vi "CSM - LogViewer2.vi"() -> ()   [LabVIEW 2017]
uses:
  Utility/_support/Periodic String Filter Level.ctl
  _jksm/_action.ctl
  Utility/Periodic String Filter Setting.ctl
  <vilib>/addons/_JKI Toolkits/State Machine/_JKI_lib_State_Machine.llb/Parse State Queue__JKI_lib_State_Machine.vi
  Communicable State Machine.lvlib
  _Shared/CSM Shared.lvlib
  _Support/csm-tool-support.lvlib
  _csmHelper/API with lvcsm Support/CSM-Helper API with lvcsm Support.lvlib
  addons/Logger/CSM File Logger.lvlib
  _ui/csm-ui-support.lvlib
  _jksm/_jkism_magic.lvlib
panel:
  out "Error(#)":i64 caption="Error(#):"
  in  "Record.Stop":bool
  in  "Record.Start":bool
  in  "Clear":bool
  in  "BackTop":bool
  in  "Toolbar.History Length(char)":i32=50000 caption="History(char)" min=1000 max=100000000 step=1
  in  "Peroid Logs":bool
  in  "Tab":T1(tab)
  out "State History":string
  out "Error History":string
  out "Broadcast Registry":string[][](table)
  out "LogInQ":i32 caption="LogInQ:"
  out "log handling Speed(#/s)":dbl caption="log handling Speed(#/s):"
  out "LogInQ change(#/s)":dbl caption="LogInQ change(#/s):"
  out "Level":T2 caption="Level:"
  in  "Stop":bool
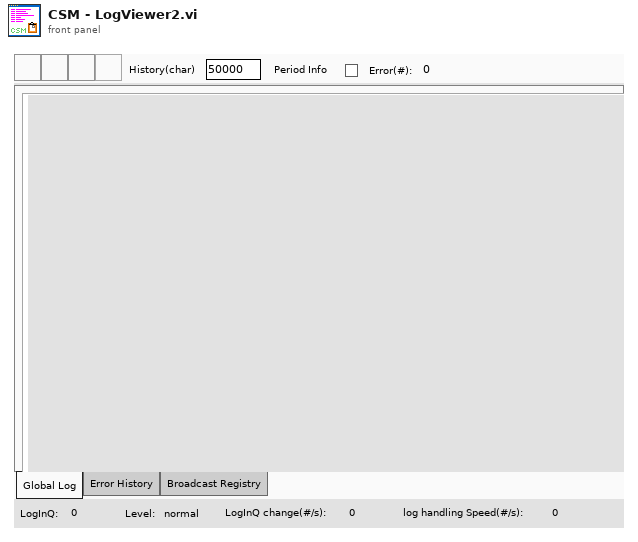
[diagram p1: front panel]
types:
  T1 = enum32{"Global Log", "Error History", "Broadcast Registry"}
  T2 = typedef "Communicable State Machine.lvlib/Periodic String Filter Level.ctl" = enum16{"normal", "L1", "L2", "L3", "L4"}
  T3 = typedef "_jkism_magic.lvlib/_action.ctl" = enum16{"Obtain", "Destroy", "Broadcast", "Post"}
  T4 = typedef "Communicable State Machine.lvlib/Periodic String Filter Setting.ctl" = cluster{"threashold(#/s)":dbl, "Check Peroid(s)":dbl}
  T5 = typedef "Communicable State Machine.lvlib/_CSM_GlobalLog_MSG.ctl" = cluster{"Name (\"\" to Use UUID)":string, "Current State":string, "Arguments":string, "Source Message":T6, "Source Module":string, "Complete(T)/Start(F)":bool, "LogType":T7, "Time Stamp":timestamp}
  T6 = typedef "Communicable State Machine.lvlib/_CSM_Response Source Message.ctl" = cluster{"‘State":string, "’Arguments":string, "’Error":errorcluster}
  T7 = typedef "Communicable State Machine.lvlib/_CSM_GlobalLog_MSG_TYPE.ctl" = enum16{"User Log", "State Change", "Status", "Interrupt", "Register", "Unregister", "Error Log", "Module Created", "Module Destroyed", "Async Message", "No-Rep Async Message", "Sync Message"}
  T8 = enum32{"Invalid", "Standard", "Closed", "Hidden", "Minimized", "Maximized"}
  T9 = enum32{"invalid app kind", "Development System", "Run Time System", "Student Edition", "Embedded LabVIEW", "Evaluation", "Custom"}
  T10 = typedef "LVPoint32TypeDef.ctl" = cluster{"Horizontal":i32, "Vertical":i32}
  T11 = cluster{"Shift":bool, "Ctrl":bool, "Alt":bool, "Cmd":bool, "Opt":bool}
  T12 = cluster{"Core":cluster{"Current VI Reference":refnum<vi>, "Close Panel on Exit?":bool}, "Toolbar.Advance":refnum<vi>[], "LoggerWatchDogQueue":refnum<queue>, "LogFile":path}
  T13 = cluster{"Current VI Reference":refnum<vi>, "Close Panel on Exit?":bool}
  T14 = typedef "Communicable State Machine.lvlib/CSM - Broadcast Message Type.ctl" = enum16{"<Null>", "Status", "Interrupt"}
  T15 = cluster{string, "Name":string, "Target CSM":string, "Target State":string, "Register Type":T14}[]
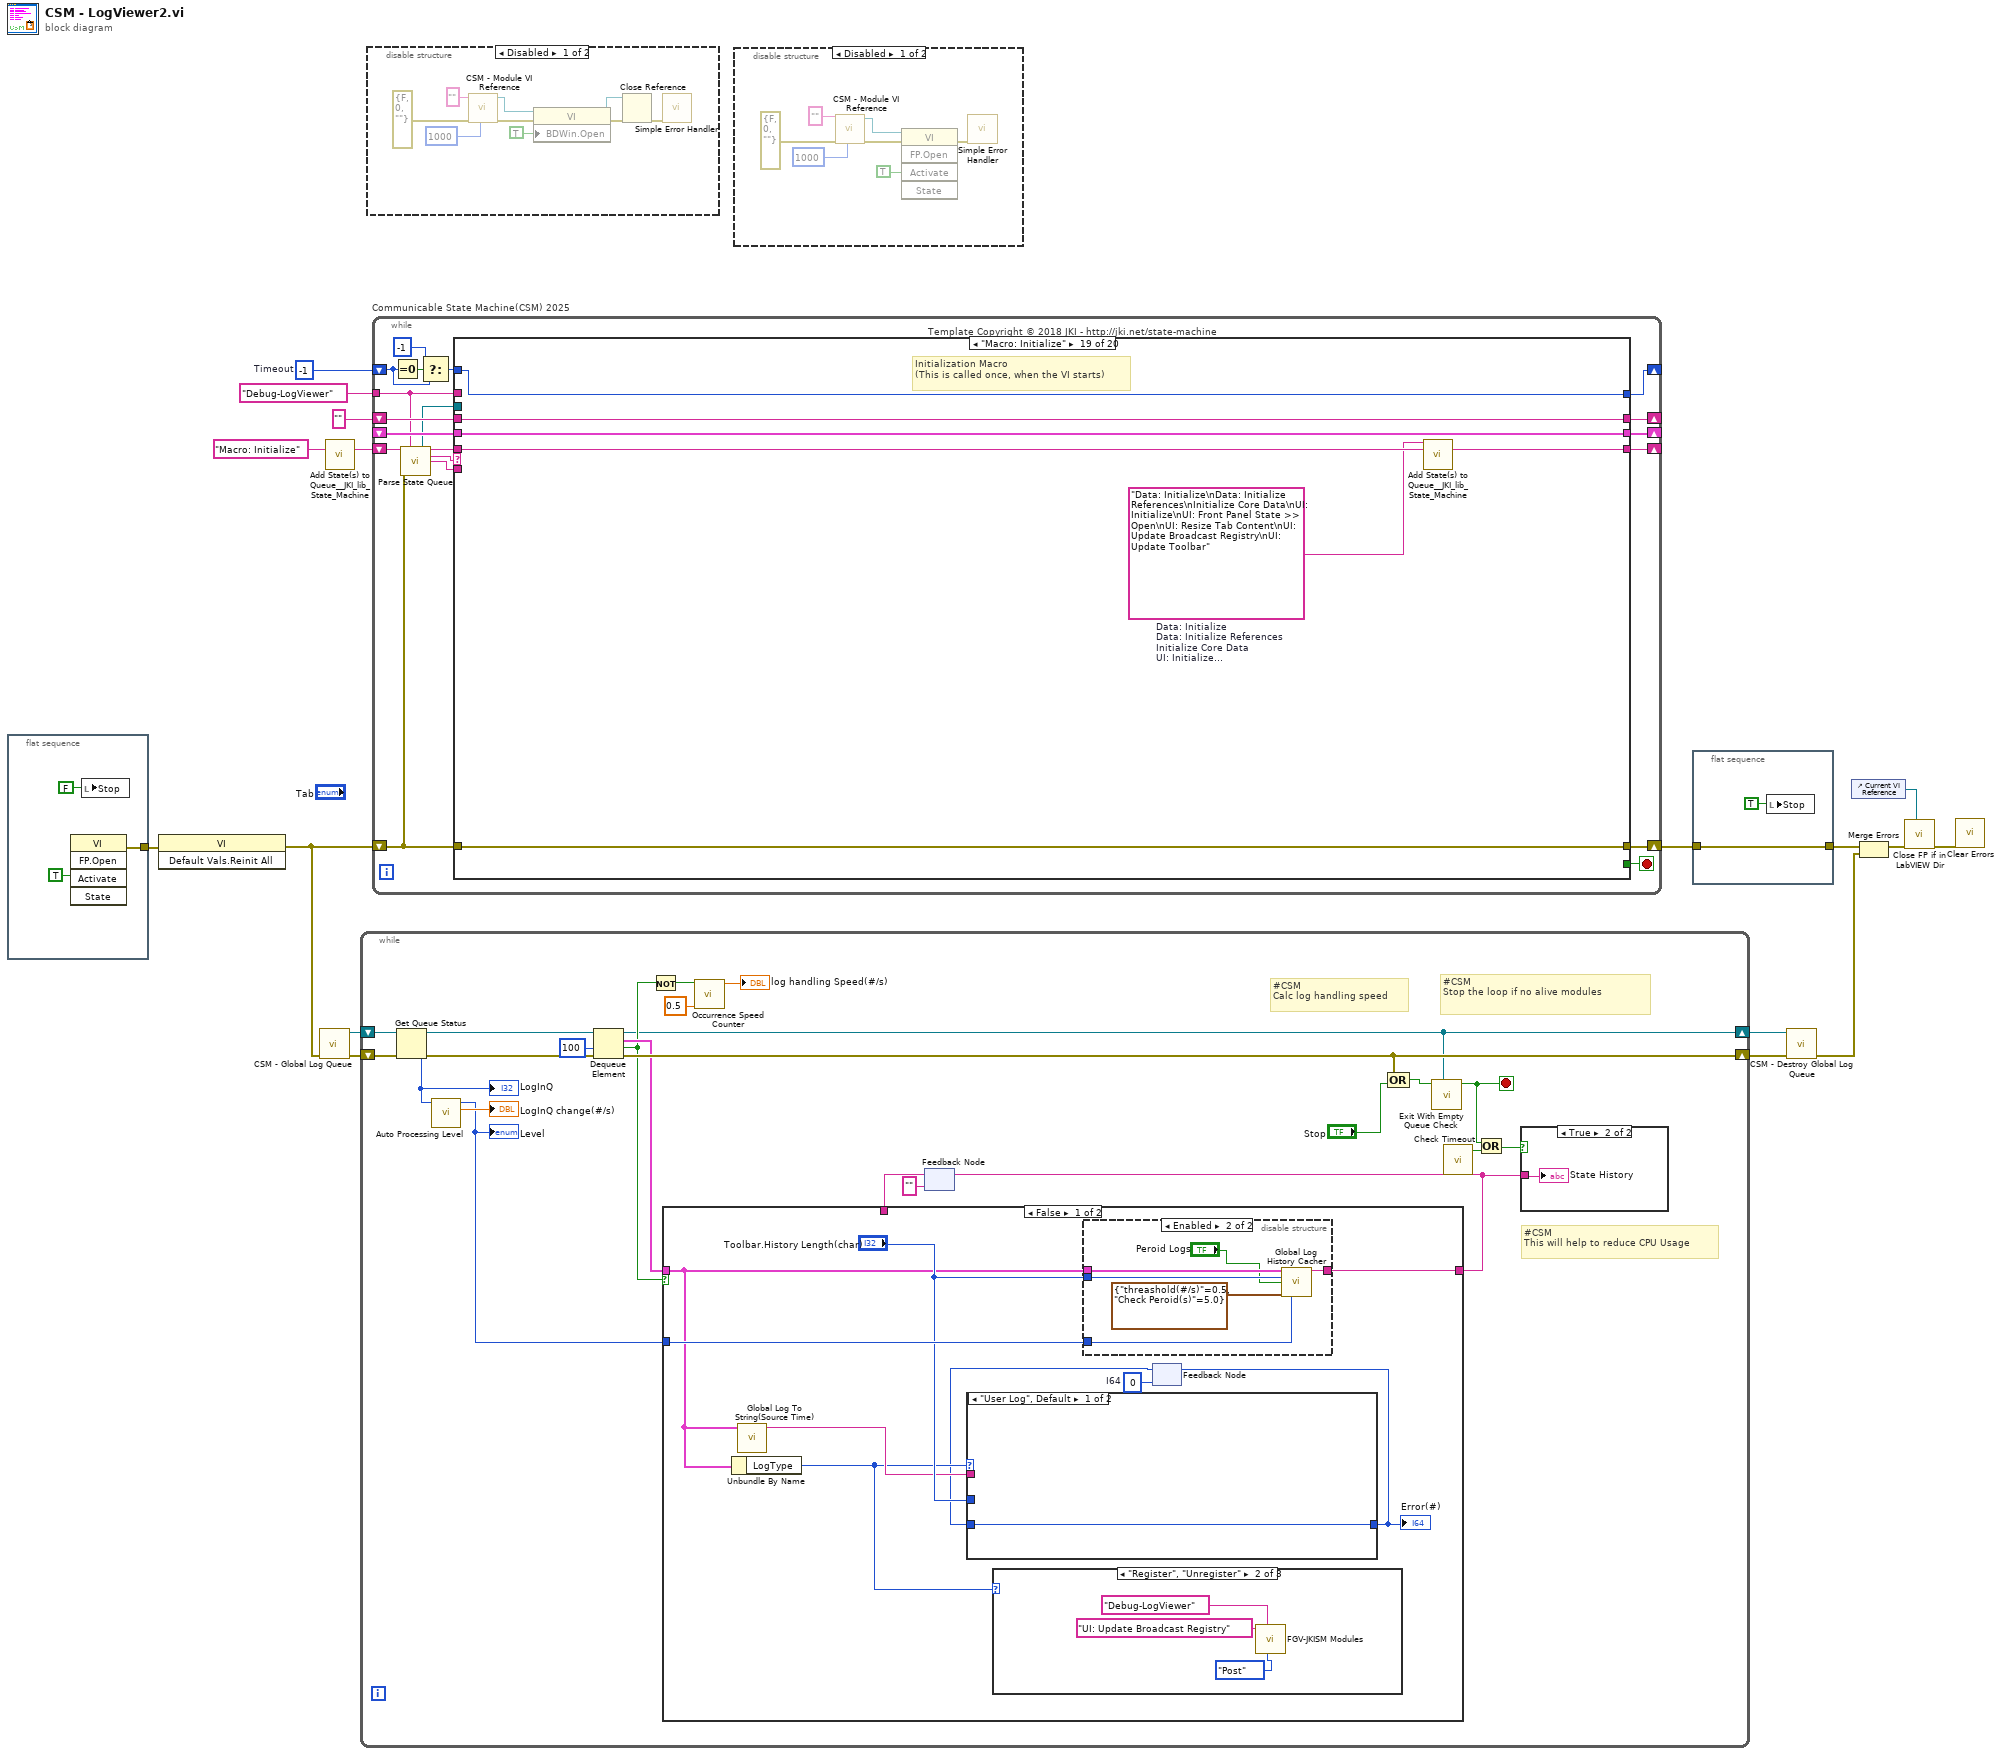
[diagram p0: block diagram]
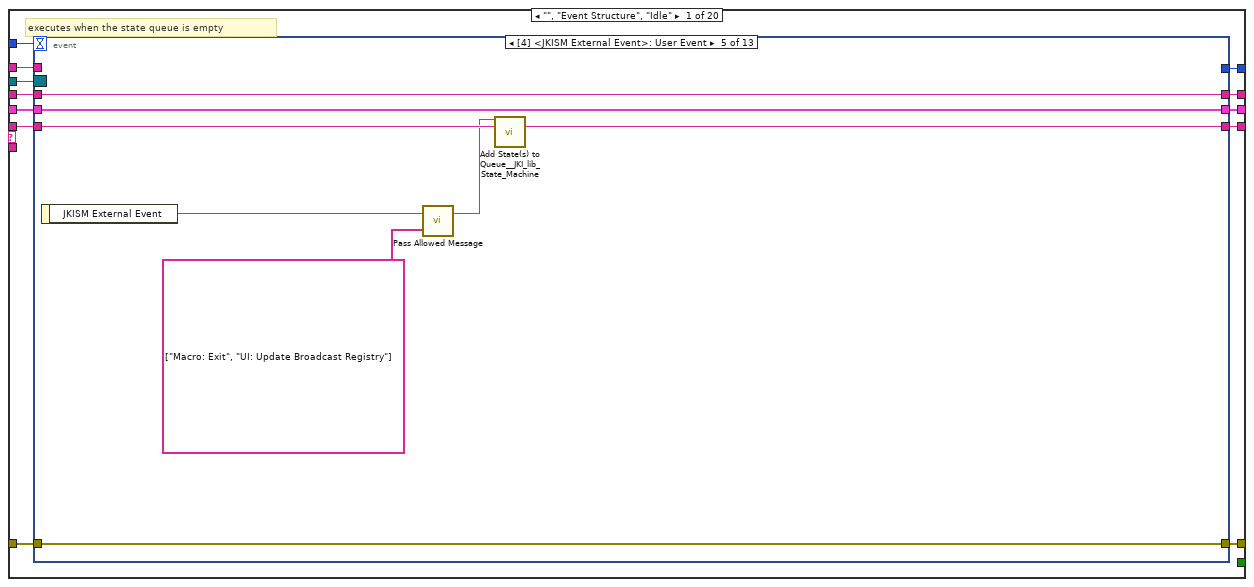
[diagram p4: hidden frame]
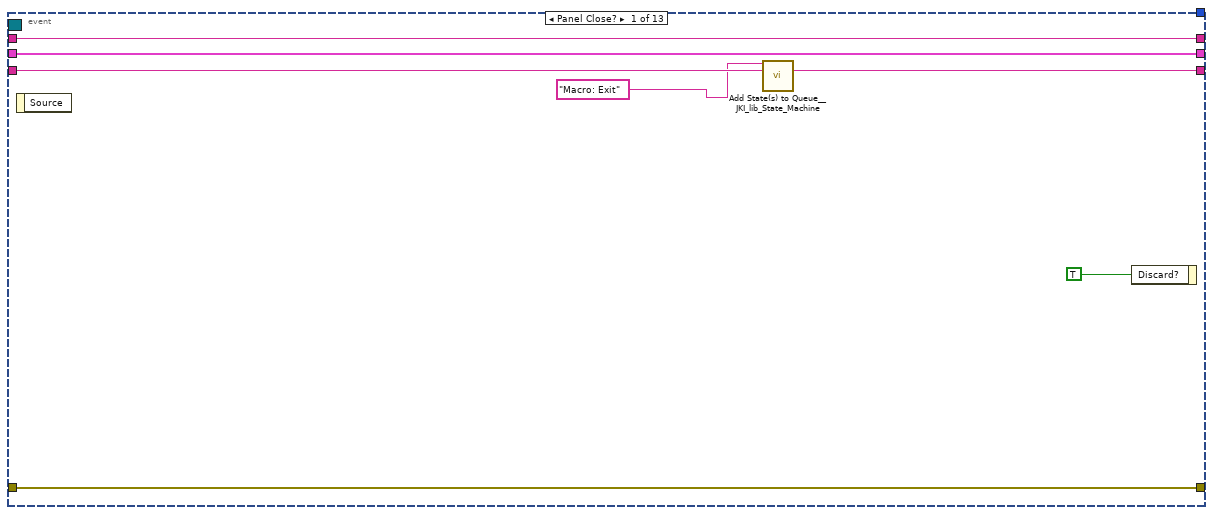
[diagram p5: hidden frame]
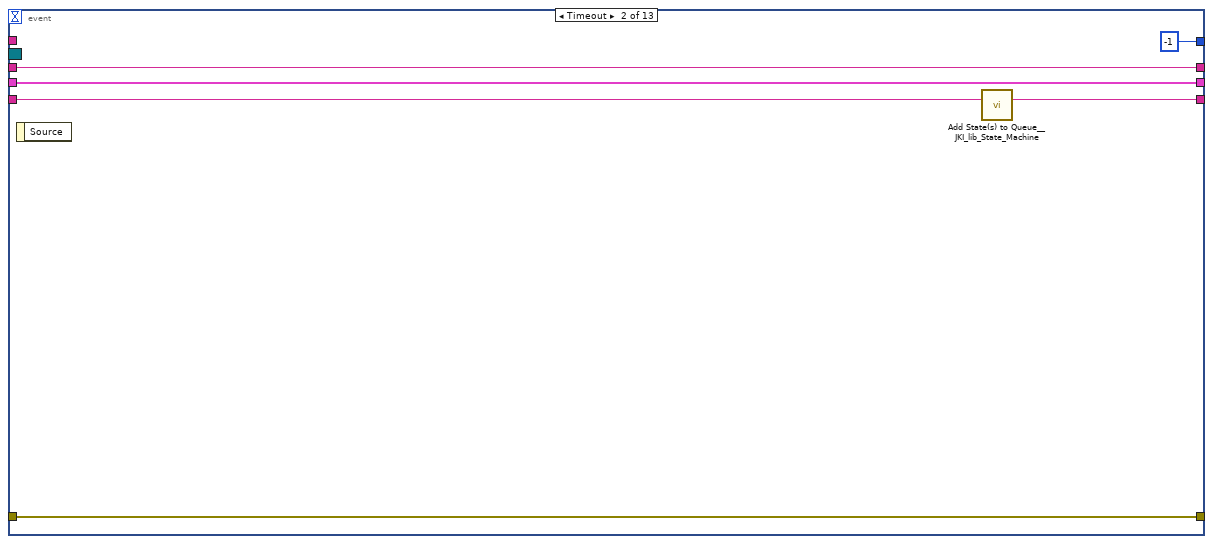
[diagram p6: hidden frame]
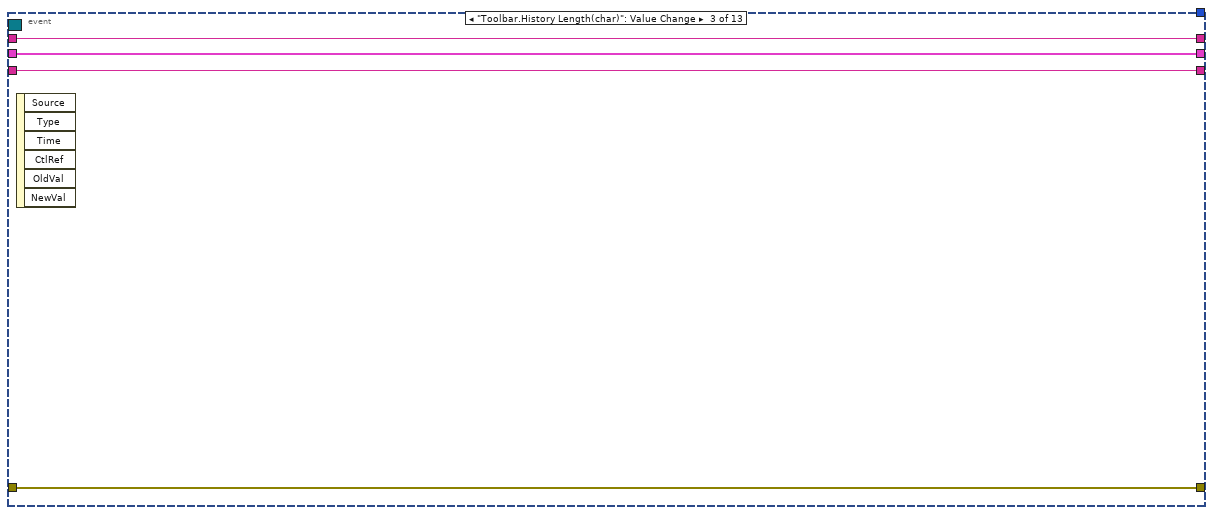
[diagram p7: hidden frame]
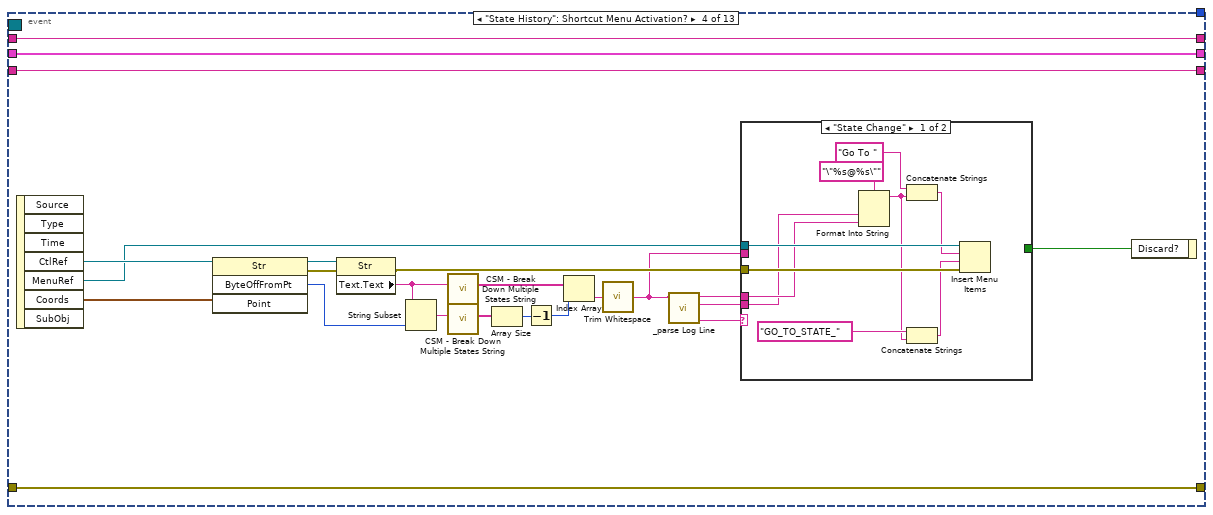
[diagram p8: hidden frame]
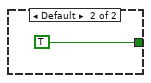
[diagram p9: hidden frame]
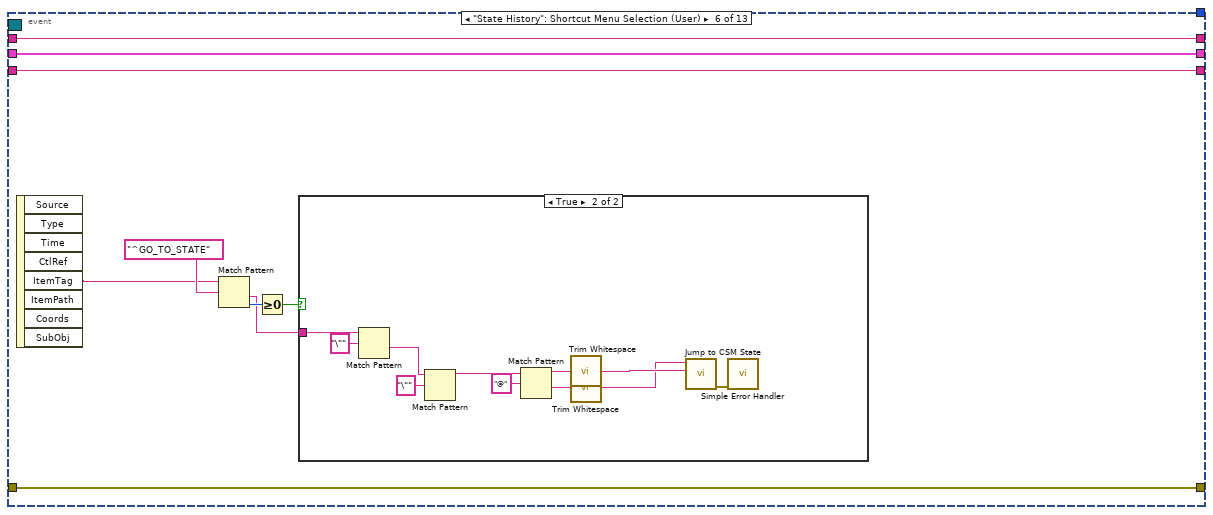
[diagram p10: hidden frame]
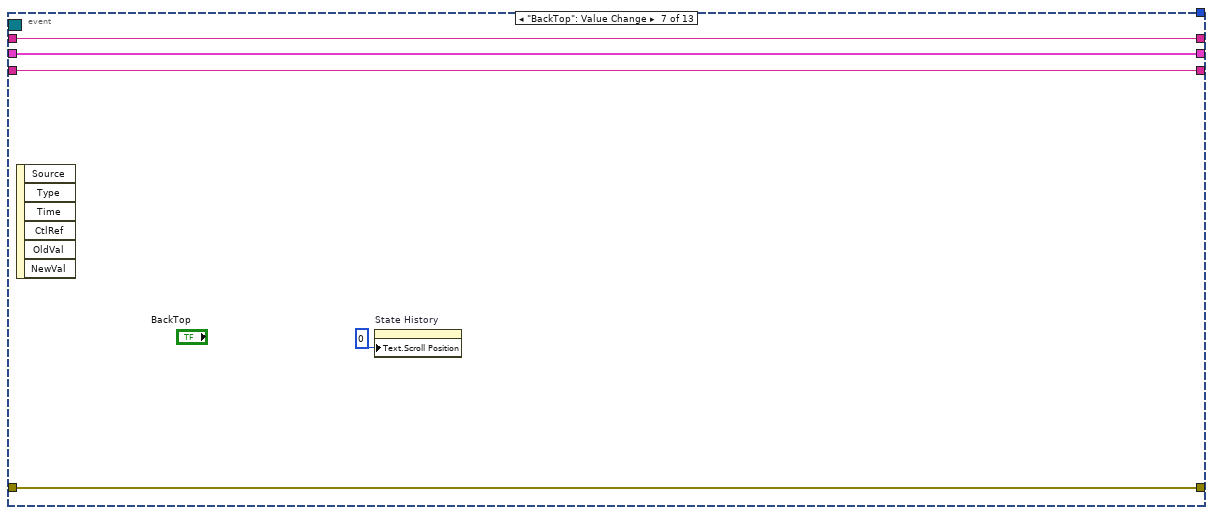
[diagram p12: hidden frame]
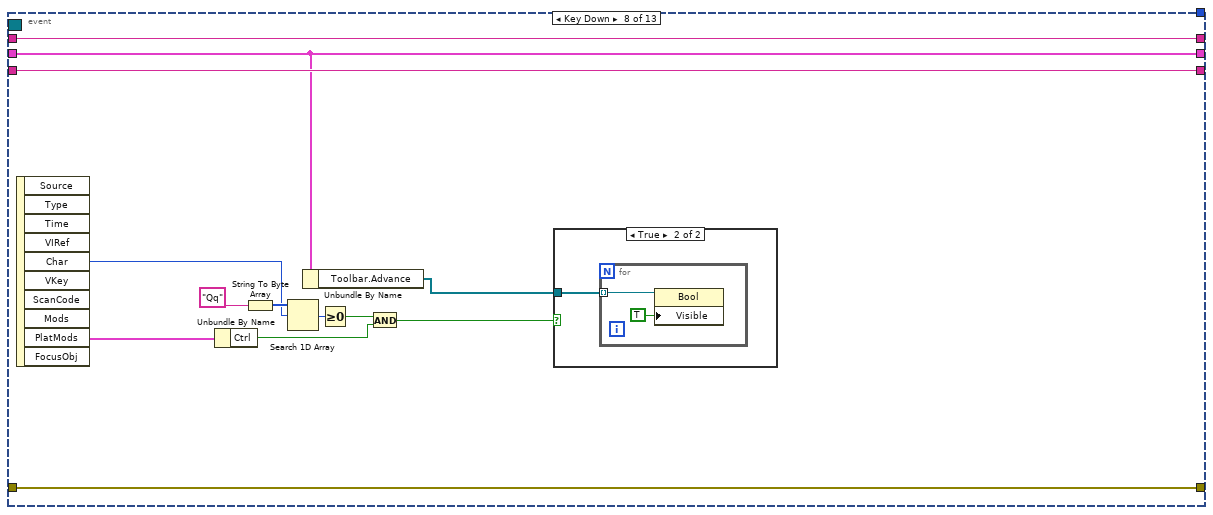
[diagram p13: hidden frame]
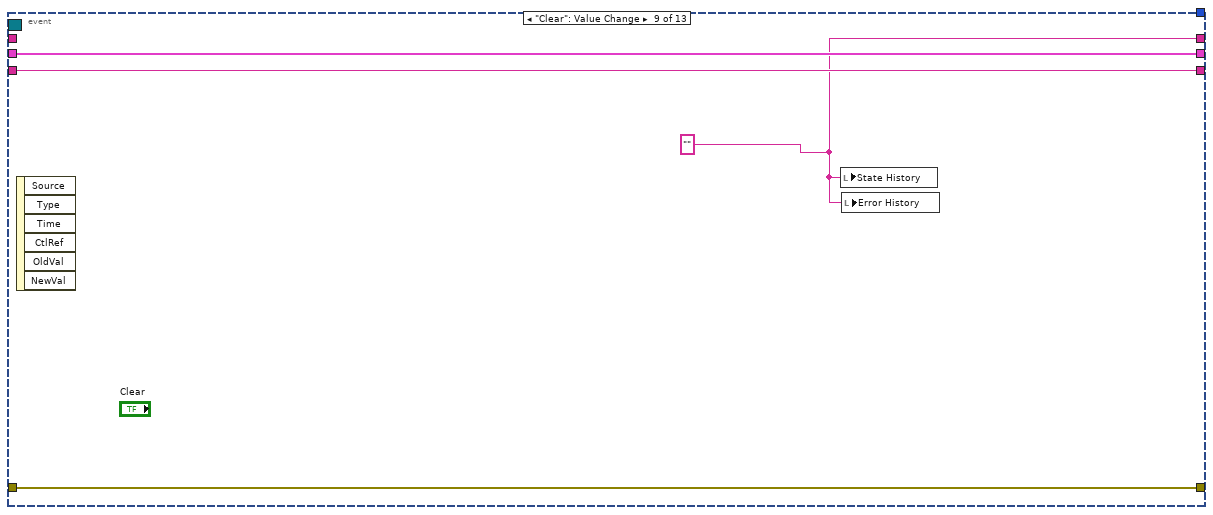
[diagram p15: hidden frame]
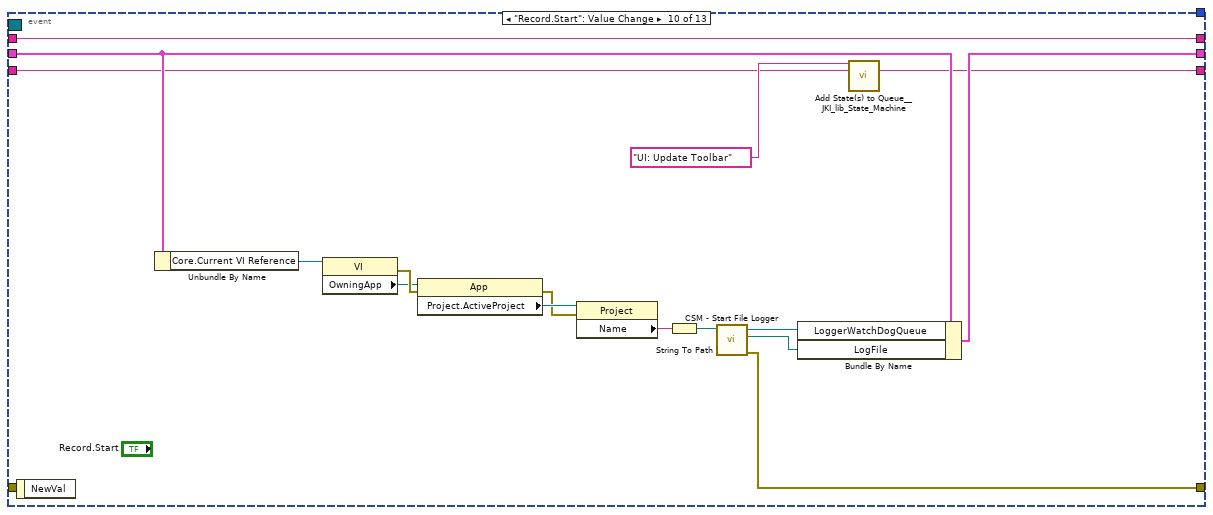
[diagram p16: hidden frame]
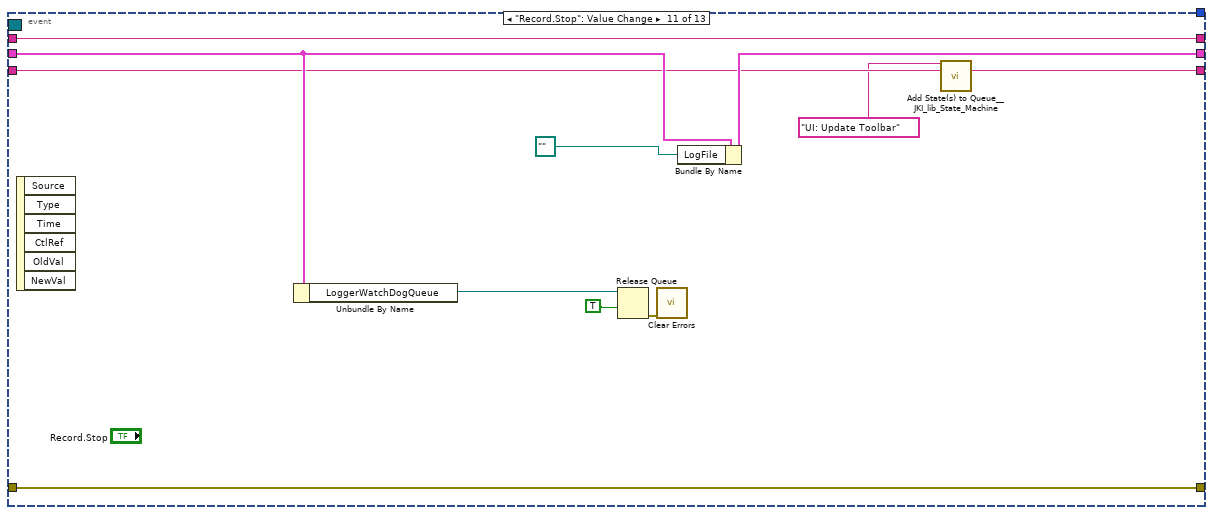
[diagram p17: hidden frame]
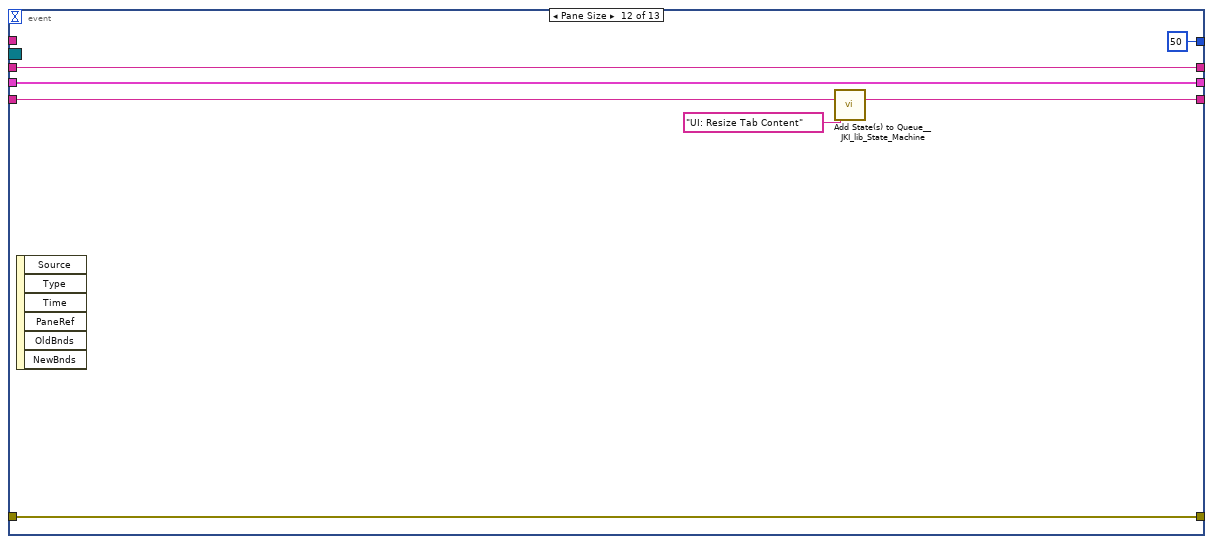
[diagram p18: hidden frame]
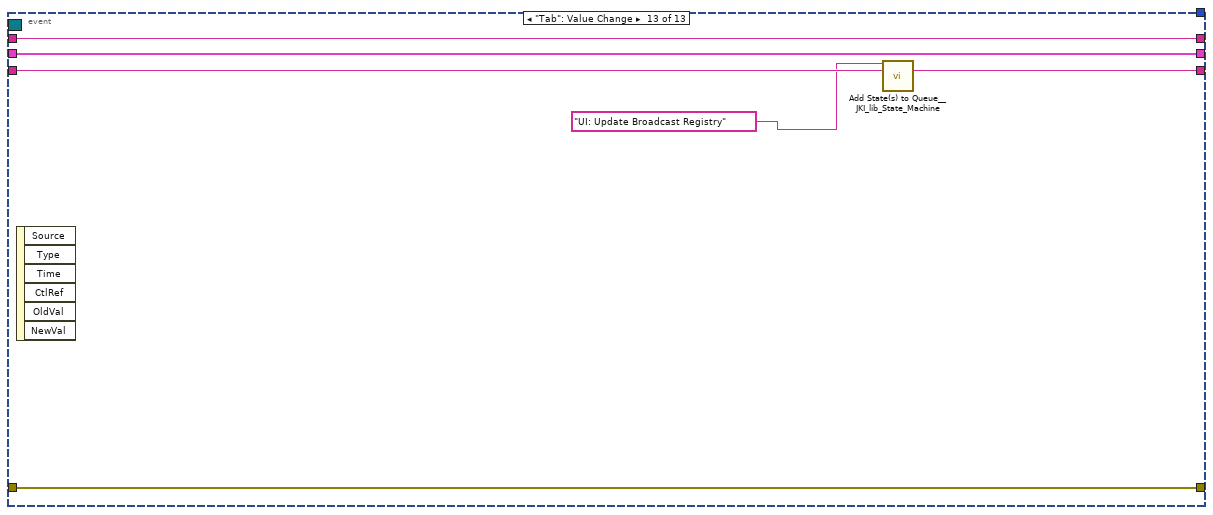
[diagram p19: hidden frame]
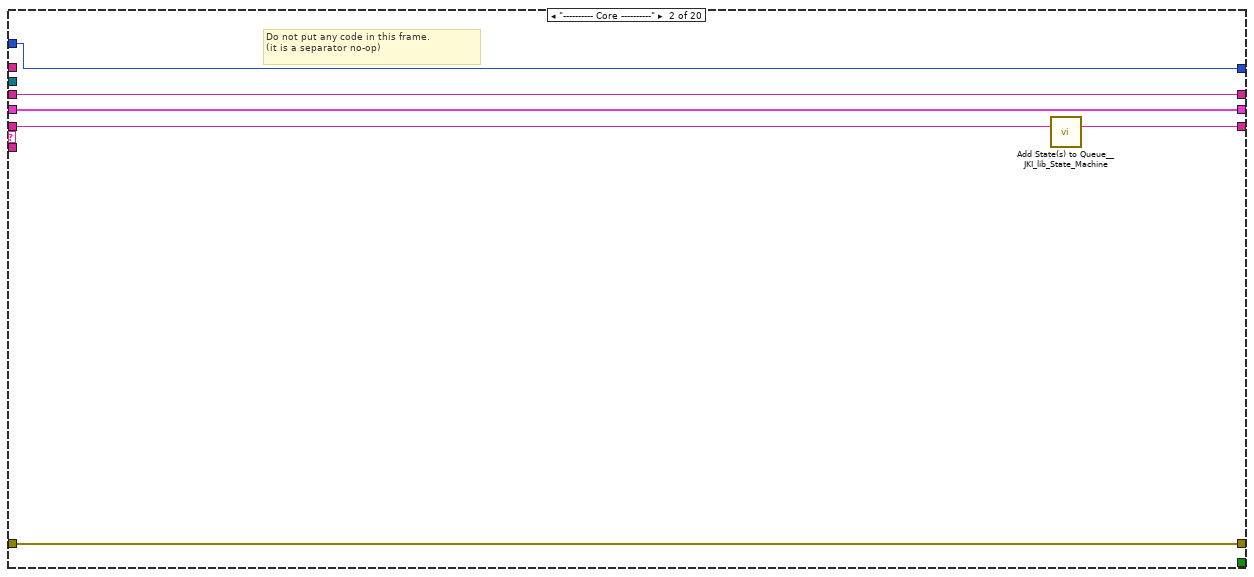
[diagram p20: hidden frame]
diagram:
  w10 = -1  # Timeout
  n1 = flat-sequence {
    tunnel: [w18] -> w6
    frame #0 {
      n2 = invoke class="VI" method="FP.Open"("Activate"=TRUE ("Activate?")) -> (error out=w18:errorcluster)  [unwired: 4 in, 4 out]
      n3 = local write "Stop"(FALSE ("Stop")) -> ()
    }
  }
  n4 = invoke class="VI" method="Default Vals.Reinit All"(error in=w6) -> (error out=w1:errorcluster)  [unwired: 2 in, 2 out]
  n5 = call "CSM - Global Log Queue.vi"("Error In"=w1) -> ("error out"=w16:errorcluster, "Global Log Queue"=w14:refnum<queue>)  [unwired: 9 in]
  n6 = call <vilib>:"Add State(s) to Queue__JKI_lib_State_Machine.vi"("State(s) in (\"\")"="Macro: Initialize") -> ("States Out"=w13:string)  [unwired: 14 in]
  n7 = while {
    shift-right: [w42] -> w17
    shift-left: w16 -> [w39]
    shift-right: [w29] -> w15
    shift-left: w14 -> [w43]
    stop <- w22 stop-if-true
    # "#CSM\nCalc log handling speed"
    # "#CSM\nStop the loop if no alive modules"
    # "#CSM\nThis will help to reduce CPU Usage"
    n8 = Get Queue Status(queue=w43, error in (no error)=w39) -> (queue out=w41:refnum<queue>, error out=w40:errorcluster, # elements in queue=w25:i32)  [unwired: 1 in, 5 out]
    "LogInQ" <- w25
    n9 = call "Auto Processing Level.vi"("#Left In Q"=w25) -> ("LogInQ Changing Speed (#/s)"=→"LogInQ change(#/s)":dbl, "Level"=w24:T2)  [unwired: 8 in, 1 out]
    "Level" <- w24
    n10 = Dequeue Element(queue=w41, timeout in ms (-1)=100, error in (no error)=w40) -> (queue out=w29:refnum<queue>, element=w38:T5, timed out?=w31:bool, error out=w42:errorcluster)
    n11 = Not(x=w31) -> (.not. x?=w30:bool)
    n12 = call "Occurrence Speed Counter.vi"("Period (0.1s)"=0.5, "Occured? (T)"=w30) -> ("Speed (#/s)"=→"log handling Speed(#/s)":dbl)  [unwired: 7 in, 2 out]
    n13 = feedback #1("" ("String Cache")) -> (w34:string)
    n14 = case shown="False" w31 {
      tunnel: w38 -> [w49 _]
      tunnel: [w52 w85] -> w35
      tunnel: w34 -> [_ w85]
      tunnel: w24 -> [w51 _]
      frame False {
        w45 = i64 0  # I64
        n15 = Unbundle By Name(w49) -> ("LogType"=w47:T7)
        n16 = call "Global Log To String(Source Time).vi"("Log"=w49) -> ("Log String"=w48:string)  [unwired: 9 in]
        n17 = case shown="\"Register\", \"Unregister\"" w47 {
          frame "User Log", Default {
          }
          frame "Register", "Unregister" {
            n18 = call "FGV-JKISM Modules.vi"("Enum"=_action."Post", "Module Name"="Debug-LogViewer" ("Current Module(\"\" to generate an ID)"), "Message"="UI: Update Broadcast Registry" ("event data")) -> ()  [unwired: 7 in, 2 out]
          }
          frame "Module Created", "Module Destroyed" {
            n19 = call "FGV-JKISM Modules.vi"("Enum"=_action."Post", "Module Name"="Debug-LogViewer" ("Current Module(\"\" to generate an ID)"), "Message"="UI: Update Broadcast Registry" ("event data")) -> ()  [unwired: 7 in, 2 out]
            n20 = call "FGV-JKISM Modules.vi"("Enum"=_action."Broadcast", "Message"="CSM: Module List Changed") -> ()  [unwired: 8 in, 2 out]
          }
        }
        n21 = disable-structure shown="Enabled" {
          disable-tunnel: w49 -> [w78 w83]
          disable-tunnel: [w76 w84] -> w52
          disable-tunnel: w51 -> [_ w82]
          disable-tunnel: "Toolbar.History Length(char)" -> [_ w80]
          frame Disabled {
            # "#CSM \nno periodical filter"
            n22 = call "Global Log To String(Source Time).vi"("Log"=w78) -> ("Log String"=w77:string)  [unwired: 9 in]
            n23 = call "String History Cacher.vi"("String"=w77) -> ("String Cache"=w76:string)  [unwired: 10 in]
          }
          frame Enabled {
            n24 = call "Global Log History Cacher.vi"("Global Log Data"=w83, "Length (10000)"=w80, "With Periodic Info? (T)"="Peroid Logs", "Settings"=T4 {"threashold(#/s)"=0.5, "Check Peroid(s)"=5.0}, "Level (Normal)"=w82) -> ("String Cache"=w84:string)  [unwired: 10 in]
          }
        }
        n25 = feedback #2(w45) -> (w44:i64)
        n26 = case shown="\"User Log\", Default" w47 {
          tunnel: w48 -> [_ w65]
          tunnel: "Toolbar.History Length(char)" -> [_ w64]
          tunnel: [w61 w63] -> w46
          tunnel: w44 -> [w61 w62]
          frame "User Log", Default {
          }
          frame "Error Log" {
            n27 = local read "Error History"() -> (w69:string)
            n28 = case shown="\"\"" w65 {
              selector: w65 -> [_ w72]
              tunnel: "\r" -> [_ w75]
              tunnel: w69 -> [w71 w74]
              tunnel: [w71 w73] -> w67
              frame "" {
              }
              frame Default {
                n29 = Concatenate Strings(w72, w75, w74) -> (w73:string)
              }
            }
            n30 = Increment(x=w62) -> (x+1=w63:i64)
            n31 = String Subset(string=w67, offset (0)=0, length (rest)=w64) -> (substring=→"Error History":string)
          }
        }
        "Error(#)" <- w46
        n32 = feedback-in #2(w46) -> ()
      }
      frame True {
      }
    }
    n33 = feedback-in #1(w35) -> ()
    n34 = Compound Arithmetic op=OR(w42, "Stop") -> (w27:bool)
    n35 = call "Exit With Empty Queue Check.vi"("Queue"=w29, "Stop"=w27) -> ("Exit"=w22:bool)  [unwired: 8 in, 1 out]
    n36 = call "Check Timeout.vi"() -> ("Timeout"=w36:bool)  [unwired: 8 in]
    n37 = Or(x=w22, y=w36) -> (x .or. y?=w28:bool)
    n38 = case shown="True" w28 {
      tunnel: w35 -> [_ w86]
      frame False {
      }
      frame True {
        "State History" <- w86
      }
    }
  }
  n39 = disable-structure shown="Disabled" {
    frame Disabled {
      n40 = call "CSM - Module VI Reference.vi"("Response Timeout (-2 Using Global Settings)"=1000 ("Response Timeout(5000 ms)"), "error in (no error)"=errorcluster {"status"=FALSE, "code"=0, "source"=""}, "CSM Name"="") -> ("error out"=w95:errorcluster, "CSM Module VIRef"=w92:refnum<vi>)  [unwired: 7 in]
      n41 = property class="VI"(reference=w92, error in=w95, "BDWin.Open"=TRUE ("Block Diagram Window:Open")) -> (reference out=w93:refnum<vi>, error out=w94:errorcluster)
      n42 = Close Reference(reference=w93, error in (no error)=w94) -> (error out=w91:errorcluster)
      n43 = call <vilib>:"Simple Error Handler.vi"("error in (no error)"=w91) -> ()  [unwired: 4 in, 5 out]
    }
    frame Enabled {
    }
  }
  n44 = while "Communicable State Machine(CSM) 2025" {
    shift-right: [w107] -> _
    shift-left: _ -> [w106]
    shift-right: [w110] -> w7
    shift-left: w1 -> [w105]
    shift-right: [w109] -> _
    shift-left: w13 -> [w111]
    tunnel: "Debug-LogViewer" ("Current Module(\"\" to generate an ID)") -> [w97]
    shift-right: [w103] -> _
    shift-left: "" ("String Cache") -> [w104]
    shift-right: [w102] -> _
    shift-left: w10 -> [w99]
    stop <- w108 stop-if-true
    # "Template Copyright © 2018 JKI - http://jki.net/state-machine"
    n45 = Equal To 0?(x=w99) -> (x = 0?=w101:bool)
    n46 = call "Parse State Queue.vi"("State Queue"=w111, "Current Module(\"\" to generate an ID)"=w97, "Error In (no error)"=w105) -> ("Event Registration Refnum"=w96:refnum<event-registration>, "Remaining States"=w113:string, "Current State"=w114:string, "Arguments"=w112:string)  [unwired: 9 in]
    n47 = Select(t=-1 ("Timeout"), s=w101, f=w99) -> (s? t:f=w100:i32)
    n48 = case shown="\"Macro: Initialize\"" w114 {
      selector: w114 -> [_ _ w279 _ _ _ _ _ _ _ _ _ _ _ _ _ _ _ _ _]
      tunnel: w113 -> [w126 w276 w283 w304 w312 w319 w325 w335 w340 w348 w354 w362 w373 w386 w457 w485 w503 w513 w520 w528]
      tunnel: w112 -> [_ _ _ _ _ _ _ _ _ _ _ _ w368 w380 _ _ _ _ _ _]
      tunnel: w106 -> [w124 w273 w281 w297 w309 w317 w322 _ w339 w343 w351 w358 w371 w382 w456 w481 w502 w510 w517 w525]
      tunnel: [w123 w274 w285 w301 errorcluster {"status"=FALSE, "code"=0, "source"=""} ("error out") w316 w323 w332 w337 w344 w352 w360 w369 w383 w458 w486 w504 w511 w518 w526] -> w110
      tunnel: w105 -> [w122 w274 w284 w301 w308 w316 w323 w332 w337 w345 w352 w360 w370 w384 w458 w486 w504 w511 w518 w526]
      tunnel: [w125 w275 w282 w303 w311 w318 w324 w334 w340 w347 w353 w361 w372 w385 w457 w485 w503 w512 w519 w527] -> w109
      tunnel: [_ _ _ _ _ TRUE _ _ _ _ _ _ _ _ _ _ _ _ _ _] -> w108
      tunnel: [w121 w273 w281 w302 w309 w317 w322 w333 w339 w343 w351 w358 w371 w382 w456 w481 w502 w510 w517 w525] -> w107
      tunnel: w100 -> [w120 w271 w277 w290 w305 w313 w320 w326 w336 w341 w349 w355 w366 w378 w452 w467 w500 w508 w514 w521]
      tunnel: w96 -> [w119 _ _ _ _ _ _ _ _ _ _ _ _ _ _ _ _ _ _ _]
      tunnel: w97 -> [w118 _ _ _ _ _ _ _ _ _ _ _ _ _ _ _ _ _ _ _]
      tunnel: w104 -> [w117 w272 w278 w291 w306 w314 w321 w330 w338 w342 w350 w359 w367 w379 w455 w484 w501 w509 w515 w522]
      tunnel: [w116 w272 w278 w291 w306 w314 w321 w330 w338 w342 w350 w359 w367 w379 w455 w484 w501 w509 w515 w522] -> w103
      tunnel: [w115 w271 w277 w290 w305 w313 w320 w326 w336 w341 w349 w355 w366 w378 w452 w467 w500 w508 w514 w521] -> w102
      frame "", "Event Structure", "Idle" {
        # "executes when the state queue is empty"
        n49 = event shown="[4] <JKISM External Event>: User Event" {
          selector: w119 -> [_ _ _ _ _ _ _ _ _ _ _ _ _]
          dyn-events: _ -> [_ _ _ _ _ _ _ _ _ _ _ _ _]
          timeout: w120 -> [_ _ _ _ _ _ _ _ _ _ _ _ _]
          tunnel: w126 -> [w133 w139 w143 w166 w181 w194 w210 w223 w230 w232 w249 w260 w266]
          tunnel: [w132 w138 w143 w166 w182 w194 w210 w223 w230 w231 w248 w261 w267] -> w125
          tunnel: w124 -> [w130 w136 w141 w164 w184 w192 w208 w213 w228 w241 w255 w263 w269]
          tunnel: [w131 w137 w142 w165 w185 w193 w209 w222 w229 w243 w257 w264 w270] -> w123
          tunnel: w122 -> [w131 w137 w142 w165 w185 w193 w209 w222 w229 _ w257 w264 w270]
          tunnel: [w130 w136 w141 w164 w184 w192 w208 w213 w228 w244 w251 w263 w269] -> w121
          tunnel: w118 -> [_ _ _ _ _ _ _ _ _ _ _ _ _]
          tunnel: w117 -> [w127 w135 w140 w163 w183 w191 w207 w221 _ w246 w256 w262 w268]
          tunnel: [w127 w135 w140 w163 w183 w191 w207 w221 w227 w246 w256 w262 w268] -> w116
          tunnel: [_ -1 ("Timeout") _ _ _ _ _ _ _ _ _ 50 ("Timeout") _] -> w115
          event Panel Close? {
            n50 = event-data() -> ()  [unwired: 1 in, 1 out]
            n51 = call <vilib>:"Add State(s) to Queue__JKI_lib_State_Machine.vi"("State(s) in Front (\"\")"="Macro: Exit", "State(s) in (\"\")"=w133) -> ("States Out"=w132:string)  [unwired: 13 in]
            n52 = event-data("Discard?"=TRUE) -> ()  [unwired: 1 in, 1 out]
          }
          event Timeout {
            n53 = event-data() -> ()  [unwired: 1 in, 1 out]
            n54 = call <vilib>:"Add State(s) to Queue__JKI_lib_State_Machine.vi"("State(s) in (\"\")"=w139) -> ("States Out"=w138:string)  [unwired: 14 in]
          }
          event "Toolbar.History Length(char)": Value Change {
            n55 = event-data() -> ()  [unwired: 1 in, 6 out]
          }
          event "State History": Shortcut Menu Activation? {
            n56 = event-data() -> ("CtlRef"=w146:refnum<vi>, "MenuRef"=w145:refnum<k9>, "Coords"=w144:T10)  [unwired: 1 in, 4 out]
            n57 = invoke class="Str" method="ByteOffFromPt"(reference=w146, "Point"=w144) -> (reference out=w162:refnum<vi>, error out=w160:errorcluster, "ByteOffFromPt"=w161:i32)  [unwired: 2 in, 1 out]
            n58 = property class="Str"(reference=w162, error in=w160) -> (error out=w152:errorcluster, "Text.Text"=w158:string)  [unwired: 1 out]
            n59 = String Subset(string=w158, length (rest)=w161) -> (substring=w159:string)  [unwired: 1 in]
            n60 = call "CSM - Break Down Multiple States String.vi"("States"=w158) -> ("Multiple States"=w157:string[])  [unwired: 10 in]
            n61 = call "CSM - Break Down Multiple States String.vi"("States"=w159) -> ("Multiple States"=w156:string[])  [unwired: 10 in]
            n62 = Array Size(array=w156) -> (size(s)=w155:i32)
            n63 = Decrement(x=w155) -> (x-1=w154:i32)
            n64 = Index Array(array=w157, index=w154) -> (element=w153:string)
            n65 = call <vilib>:"Trim Whitespace.vi"("string"=w153) -> ("trimmed string"=w151:string)  [unwired: 1 in]
            n66 = call "_parse Log Line.vi"("String"=w151) -> ("LogType"=w150:string, "State"=w148:string, "CSM"=w149:string)  [unwired: 8 in]
            n67 = case shown="\"State Change\"" w150 {
              tunnel: w145 -> [w176 _]
              tunnel: w151 -> [_ _]
              tunnel: w152 -> [w174 _]
              tunnel: [_ TRUE] -> w147
              tunnel: w149 -> [w172 _]
              tunnel: w148 -> [w171 _]
              frame "State Change" {
                n68 = Format Into String(format string="\"%s@%s\"", w171, w172) -> (resulting string=w167:string)  [unwired: 2 in, 1 out]
                n69 = Concatenate Strings("Go To " ("format string"), w167) -> (w170:string)
                n70 = Concatenate Strings("GO_TO_STATE_" ("item tags"), w167) -> (w168:string)
                n71 = Insert Menu Items(6:w174, 7:w168, 8:w170, 9:w176) -> ()  [unwired: 2 in, 3 out]
              }
              frame Default {
              }
            }
            n72 = event-data("Discard?"=w147) -> ()  [unwired: 1 in, 1 out]
          }
          event User Event {
            n73 = event-data() -> ("JKISM External Event"=w179:string)  [unwired: 1 in]
            n74 = call "Pass Allowed Message.vi"("Allowed Message"=string[] ["Macro: Exit", "UI: Update Broadcast Registry"] ("1D array"), "JKISM External Event"=w179) -> ("States"=w180:string)  [unwired: 1 in]
            n75 = call <vilib>:"Add State(s) to Queue__JKI_lib_State_Machine.vi"("State(s) in Front (\"\")"=w180, "State(s) in (\"\")"=w181) -> ("States Out"=w182:string)  [unwired: 13 in]
          }
          event "State History": Shortcut Menu Selection (User) {
            n76 = event-data() -> ("ItemTag"=w186:string)  [unwired: 1 in, 7 out]
            n77 = Match Pattern(string=w186, regular expression="^GO_TO_STATE") -> (after substring=w187:string, offset past match=w189:i32)  [unwired: 1 in, 2 out]
            n78 = Greater Or Equal To 0?(x=w189) -> (x >= 0?=w188:bool)
            n79 = case shown="True" w188 {
              tunnel: w187 -> [_ w205]
              frame False {
              }
              frame True {
                n80 = Match Pattern(string=w205, regular expression="\"") -> (after substring=w202:string)  [unwired: 1 in, 3 out]
                n81 = Match Pattern(string=w202, regular expression="\"") -> (before substring=w201:string)  [unwired: 1 in, 3 out]
                n82 = Match Pattern(string=w201, regular expression="@") -> (before substring=w199:string, after substring=w198:string)  [unwired: 1 in, 2 out]
                n83 = call <vilib>:"Trim Whitespace.vi"("string"=w199) -> ("trimmed string"=w197:string)  [unwired: 1 in]
                n84 = call <vilib>:"Trim Whitespace.vi"("string"=w198) -> ("trimmed string"=w196:string)  [unwired: 1 in]
                n85 = call "Jump to CSM State.vi"("State"=w197, "Name"=w196) -> ("error out"=w195:errorcluster)  [unwired: 9 in]
                n86 = call <vilib>:"Simple Error Handler.vi"("error in (no error)"=w195) -> ()  [unwired: 4 in, 5 out]
              }
            }
          }
          event "BackTop": Value Change {
            n87 = event-data() -> ()  [unwired: 1 in, 6 out]
            n88 = property on="State History" class="Str"("Text.Scroll Position"=u32 0) -> ()  [unwired: 2 in, 2 out]
          }
          event Key Down {
            n89 = event-data() -> ("Char"=w211:i16, "PlatMods"=w216:T11)  [unwired: 1 in, 8 out]
            n90 = Unbundle By Name(w216) -> ("Ctrl"=w215:bool)
            n91 = String To Byte Array(string="Qq") -> (unsigned byte array=w218:u8[])
            n92 = Search 1D Array(1D array=w218, element=w211) -> (index of element=w219:i32)  [unwired: 1 in]
            n93 = Unbundle By Name(w213) -> ("Toolbar.Advance"=w212:refnum<vi>[])
            n94 = Greater Or Equal To 0?(x=w219) -> (x >= 0?=w220:bool)
            n95 = And(x=w220, y=w215) -> (x .and. y?=w214:bool)
            n96 = case shown="True" w214 {
              tunnel: w212 -> [_ w224]
              frame False {
              }
              frame True {
                n97 = for {
                  tunnel: w224 -> [w226] mode=indexing
                  n98 = property class="Bool"(reference=w226, "Visible"=TRUE) -> ()  [unwired: 1 in, 2 out]
                }
              }
            }
          }
          event "Clear": Value Change {
            w227 = "" ("String Cache")
            n99 = event-data() -> ()  [unwired: 1 in, 6 out]
            n100 = local write "State History"(w227) -> ()
            n101 = local write "Error History"(w227) -> ()
          }
          event "Record.Start": Value Change {
            n102 = event-data() -> ()  [unwired: 1 in, 1 out]
            n103 = Unbundle By Name(w241) -> ("Core.Current VI Reference"=w240:refnum<vi>)
            n104 = property class="VI"(reference=w240) -> (error out=w239:errorcluster, "OwningApp"=w238:refnum<vi>)  [unwired: 1 in, 1 out]
            n105 = property class="App"(reference=w238, error in=w239) -> (error out=w236:errorcluster, "Project.ActiveProject"=w237:refnum<vi>)  [unwired: 1 out]
            n106 = property class="Project"(reference=w237, error in=w236) -> ("Name"=w235:string)  [unwired: 2 out]
            n107 = String To Path(string=w235) -> (path=w234:path)
            n108 = call "CSM - Start File Logger.vi"("Log File Path"=w234) -> ("error out"=w243:errorcluster, "Log File"=w242:path, "Watchdog Queue"=w245:refnum<queue>)  [unwired: 8 in]
            n109 = Bundle By Name(cluster=w241, "LoggerWatchDogQueue"=w245, "LogFile"=w242) -> (w244:T12)
            n110 = call <vilib>:"Add State(s) to Queue__JKI_lib_State_Machine.vi"("State(s) in Front (\"\")"="UI: Update Toolbar" ("State(s) in Front (\"\")"), "State(s) in (\"\")"=w232) -> ("States Out"=w231:string)  [unwired: 13 in]
          }
          event "Record.Stop": Value Change {
            n111 = event-data() -> ()  [unwired: 1 in, 6 out]
            n112 = Unbundle By Name(w255) -> ("LoggerWatchDogQueue"=w254:refnum<queue>)
            n113 = Release Queue(queue=w254, force destroy? (F)=TRUE) -> (error out=w252:errorcluster)  [unwired: 1 in, 2 out]
            n114 = call <vilib>:"Clear Errors.vi"("error in (no error)"=w252) -> ()  [unwired: 5 in, 2 out]
            n115 = Bundle By Name(cluster=w255, "LogFile"=path "") -> (w251:T12)
            n116 = call <vilib>:"Add State(s) to Queue__JKI_lib_State_Machine.vi"("State(s) in Front (\"\")"="UI: Update Toolbar" ("State(s) in Front (\"\")"), "State(s) in (\"\")"=w249) -> ("States Out"=w248:string)  [unwired: 13 in]
          }
          event Pane Size {
            n117 = event-data() -> ()  [unwired: 1 in, 6 out]
            n118 = call <vilib>:"Add State(s) to Queue__JKI_lib_State_Machine.vi"("State(s) in (\"\")"=w260, "State(s) at Back (\"\")"="UI: Resize Tab Content" ("State(s) in Front (\"\")")) -> ("States Out"=w261:string)  [unwired: 13 in]
          }
          event "Tab": Value Change {
            n119 = event-data() -> ()  [unwired: 1 in, 6 out]
            n120 = call <vilib>:"Add State(s) to Queue__JKI_lib_State_Machine.vi"("State(s) in Front (\"\")"="UI: Update Broadcast Registry" ("State(s) in Front (\"\")"), "State(s) in (\"\")"=w266) -> ("States Out"=w267:string)  [unwired: 13 in]
          }
        }
      }
      frame "---------- Core ----------" {
        # "Do not put any code in this frame.\n(it is a separator no-op)"
        n121 = call <vilib>:"Add State(s) to Queue__JKI_lib_State_Machine.vi"("State(s) in (\"\")"=w276) -> ("States Out"=w275:string)  [unwired: 14 in]
      }
      frame Default {
        w288 = 42 items=["No error", "Argument error", "Memory is full", "Out of zone", "End of file", "File already open", "Generic file I/O error", "File not found", "File permission error", "Disk is full", "Duplicate path", "Too many files open", "System feature not enabled", "Resource file not found", "Cannot add resource", "Resource not found", "Image not found", "Image memory error", "Pen does not exist", "Config type invalid", "Config token not found", "Config parse error", "Config memory error", "Bad external code format", "Bad external code offset", "External code not present", "Null window", "Destroy window error", "Null menu", "Print aborted", "Bad print record", "Print driver error", "Windows error during printing", "Memory error during printing", "Print dialog error", "Generic print error", "Invalid device refnum", "Device not found", "Device parameter error", "Device unit error", "Cannot open device", "Device call aborted", "Generic error", "Cancelled by user", "Object ID too low", "Object ID too high", "Object not in heap", "Unknown heap", "Unknown object (invalid DefProc)", "Unknown object (DefProc not in table)", "Message out of range", "Invalid (null) method", "Unknown message", "Manager call not supported", "Bad address", "Network operation in progress", "Network operation timed out", "Connection is busy", "Network attribute not supported", "Network error", "Address in use", "System out of memory", "Connection aborted", "Connection refused", "Not connected", "Already connected", "Connection closed", "Initialization error (interapplication manager)", "Bad occurrence", "Wait on unbound occurrence handler", "Occurrence queue overflow", "Datalog type conflict", "Unused", "Unrecognized type (interapplication manager)", "Memory corrupt", "Failed to make temporary DLL", "Old CIN version", "Drag socket not found", "Failed to load drop-object", "Failed to register OLE object", "Failed to release OLE object", "Format specifier type mismatch", "Unknown format specifier", "Too few format specifiers", "Too many format specifiers", "Scan failed", "Newer CIN version", "Error converting to variant", "Runtime menu error", "Password tampered", "Variant attribute not found", "Incompatible variant data type", "Event data is not available", "Event Store is not present", "Occurrence is not found", "Event Queue is not created", "Event info is not available", "Refnum passed is NULL", "Error retrieving Class GUID", "Error retrieving CoClass GUID", "Error retrieving TypeLib GUID.", "Bad built application magic bytes.", "Specific driver is different from the specific driver associated with the Logical Name.", "There is no session opened to the class driver.", "Max Error", "MAX - Error with config objects", "MAX - Error loading configuration", "MAX - Group not supported"]
        # "Current State"
        # "Do not delete, rename, or modify this frame.\n(this is used to capture unhandled states and typos)"
        # "Handle mistyped state name (developer tool)"
        n122 = Format Into String(format string="Software Exception: Unhandled State \"%s\"." ("message"), error in=w284, w279) -> (resulting string=w287:string, error out=w286:errorcluster)  [unwired: 1 in]
        n123 = call <vilib>:"Error Cluster From Error Code.vi"("show call chain? (False)"=TRUE, "error in (no error)"=w286, "error message (\"\")"=w287, "error code (0)"=w288) -> ("error out"=w285:errorcluster)  [unwired: 5 in]
        n124 = call <vilib>:"Add State(s) to Queue__JKI_lib_State_Machine.vi"("State(s) in (\"\")"=w283) -> ("States Out"=w282:string)  [unwired: 14 in]
      }
      frame "Initialize Core Data" {
        # "Do not delete, rename, or modify this frame.\n(this is used to determine panel behavior on exit)"
        # "originally closed?"
        # "exe?"
        # "If panel starts closed or is an EXE, then close it when we exit"
        n125 = property class="VI"() -> ("FP.State"=w294:T8)  [unwired: 2 in, 2 out]
        n126 = property class="App"() -> ("App.Kind"=w300:T9)  [unwired: 2 in, 2 out]
        n127 = control-ref of="Current VI Reference"() -> (w295:refnum<vi>)
        n128 = Equal?(x=w294, y=T8."Closed" ("Front Panel Window:State")) -> (x = y?=w292:bool)
        n129 = Equal?(x=w300, y=T9."Run Time System" ("Application:Kind")) -> (x = y?=w298:bool)
        n130 = Or(x=w292, y=w298) -> (x .or. y?=w296:bool)
        n131 = Bundle By Name(cluster=w297, "Core.Current VI Reference"=w295, "Core.Close Panel on Exit?"=w296) -> (w302:T12)
        n132 = call <vilib>:"Add State(s) to Queue__JKI_lib_State_Machine.vi"("State(s) in (\"\")"=w304) -> ("States Out"=w303:string)  [unwired: 14 in]
      }
      frame "Error Handler" {
        # "Unhandled Error -- Display it"
        # "Handle any errors here.\nYou can also output any states to clean-up after errors occur"
        # "Clear error"
        n133 = call <vilib>:"General Error Handler.vi"("error in (no error)"=w308) -> ()  [unwired: 10 in, 5 out]
        n134 = call <vilib>:"Add State(s) to Queue__JKI_lib_State_Machine.vi"("State(s) in Front (\"\")"="/* Post Error States", "State(s) in (\"\")"=w312) -> ("States Out"=w311:string)  [unwired: 13 in]
      }
      frame "Exit" {
        # "Do not put any code in this frame.\n(No errors that occur here will be handled.)"
        n135 = call <vilib>:"Add State(s) to Queue__JKI_lib_State_Machine.vi"("State(s) in (\"\")"=w319) -> ("States Out"=w318:string)  [unwired: 14 in]
      }
      frame "---------- Data ----------" {
        # "Do not put any code in this frame.\n(It is a separator no-op. You can make a copy of this frame to create a new Data frame)"
        n136 = call <vilib>:"Add State(s) to Queue__JKI_lib_State_Machine.vi"("State(s) in (\"\")"=w325) -> ("States Out"=w324:string)  [unwired: 14 in]
      }
      frame "Data: Initialize" {
        w327 = refnum<queue> refnum  # LoggerWatchDogQueue
        w328 = path ""  # LogFile
        w329 = refnum<vi>[] []  # Toolbar.Advance
        w331 = T13 {"Current VI Reference"=refnum, "Close Panel on Exit?"=FALSE}  # Core
        # "Data names and types of shift register data are defined by this bundle."
        # "Initialize the shift-register data, here.\n(data names are defined by what you wire into the bundle function)"
        n137 = Bundle("Core"=w331, "Toolbar.Advance"=w329, "LoggerWatchDogQueue"=w327, "LogFile"=w328) -> (w333:T12)  [unwired: 1 in]
        n138 = call <vilib>:"Add State(s) to Queue__JKI_lib_State_Machine.vi"("State(s) in (\"\")"=w335) -> ("States Out"=w334:string)  [unwired: 14 in]
      }
      frame "Data: Initialize References" {
      }
      frame "Data: Cleanup" {
        # "Cleanup any data and references, here.\n(this is called automatically, by the Macro: Exit)"
        n139 = Unbundle By Name(w343) -> ("Core.Current VI Reference"=w346:refnum<vi>)
        n140 = Close Reference(reference=w346, error in (no error)=w345) -> (error out=w344:errorcluster)
        n141 = call <vilib>:"Add State(s) to Queue__JKI_lib_State_Machine.vi"("State(s) in (\"\")"=w348) -> ("States Out"=w347:string)  [unwired: 14 in]
      }
      frame "---------- UI ----------" {
        # "Do not put any code in this frame.\n(It is a separator no-op. You can make a copy of this frame to create a new UI frame)"
        n142 = call <vilib>:"Add State(s) to Queue__JKI_lib_State_Machine.vi"("State(s) in (\"\")"=w354) -> ("States Out"=w353:string)  [unwired: 14 in]
      }
      frame "UI: Initialize" {
        # "Initialize the User Interface, here.\n(this is called automatically, by the Macro: Init)"
        n143 = Unbundle By Name(w358) -> ("Toolbar.Advance"=w357:refnum<vi>[])
        n144 = disable-structure shown="Disabled" {
          disable-tunnel: w357 -> [w363 _]
          frame Disabled {
            n145 = for {
              tunnel: w363 -> [w365] mode=indexing
              n146 = property class="Bool"(reference=w365, "Visible"=FALSE) -> ()  [unwired: 1 in, 2 out]
            }
          }
          frame Enabled {
          }
        }
        n147 = local write "Peroid Logs"(TRUE ("Filter Peroid Logs")) -> ()
        n148 = call <vilib>:"Add State(s) to Queue__JKI_lib_State_Machine.vi"("State(s) in (\"\")"=w362) -> ("States Out"=w361:string)  [unwired: 14 in]
      }
      frame "UI: Cursor Set" {
        # "Argument"
        # "Set and Unset Cursor Busy.\n(Usage: \"UI: Cursor Set >> Busy|Idle\")"
        n149 = case shown="\"Idle\", Default" w368 {
          tunnel: w370 -> [w375 w377]
          tunnel: [w374 w376] -> w369
          frame "Idle", Default {
            n150 = call <vilib>:"Unset Busy.vi"("error in (no error)"=w375) -> ("error out"=w374:errorcluster)  [unwired: 10 in]
          }
          frame "Busy" {
            n151 = call <vilib>:"Set Busy.vi"("error in (no error)"=w377) -> ("error out"=w376:errorcluster)  [unwired: 9 in, 1 out]
          }
        }
        n152 = call <vilib>:"Add State(s) to Queue__JKI_lib_State_Machine.vi"("State(s) in (\"\")"=w373) -> ("States Out"=w372:string)  [unwired: 14 in]
      }
      frame "UI: Front Panel State" {
        # "Argument"
        # "Set Front Panel Open or Closed\n(Usage: \"UI: Front Panel State >> Open|Close\")"
        n153 = Unbundle By Name(w382) -> ("Core.Current VI Reference"=w381:refnum<vi>)
        n154 = case shown="\"Minimize\", \"Minimized\"" w380 {
          tunnel: w384 -> [w392 w407 w418 w431 w444]
          tunnel: [w394 w408 w420 w433 w446] -> w383
          tunnel: w381 -> [w393 w405 w419 w432 w445]
          frame "Open", "Standard", Default {
            w387 = T8."Standard" ("State")
            n155 = property class="VI"(reference=w393, error in=w392) -> (reference out=w390:refnum<vi>, error out=w391:errorcluster, "FP.State"=w389:T8)
            n156 = Not Equal?(x=w389, y=w387) -> (x != y?=w388:bool)
            n157 = case shown="True" w388 {
              tunnel: [w398 w400] -> w394
              tunnel: w391 -> [w397 w400]
              tunnel: w390 -> [w396 _]
              tunnel: w387 -> [w395 _]
              frame True {
                n158 = invoke class="VI" method="FP.Open"(reference=w396, error in=w397, "Activate"=TRUE, "State"=w395) -> (error out=w398:errorcluster)  [unwired: 1 in, 4 out]
              }
              frame False {
              }
            }
          }
          frame "Close", "Closed" {
            n159 = property class="VI"(reference=w405, error in=w407) -> (reference out=w404:refnum<vi>, error out=w406:errorcluster, "FP.State"=w402:T8)
            n160 = Not Equal?(x=w402, y=T8."Closed" ("Front Panel Window:State")) -> (x != y?=w401:bool)
            n161 = case shown="True" w401 {
              tunnel: [w409 w412] -> w408
              tunnel: w406 -> [w409 w411]
              tunnel: w404 -> [_ w410]
              frame False {
              }
              frame True {
                n162 = invoke class="VI" method="FP.Close"(reference=w410, error in=w411) -> (error out=w412:errorcluster)  [unwired: 1 in, 2 out]
              }
            }
          }
          frame "Hidden", "Hide" {
            w413 = T8."Hidden" ("State")
            n163 = property class="VI"(reference=w419, error in=w418) -> (reference out=w416:refnum<vi>, error out=w417:errorcluster, "FP.State"=w415:T8)
            n164 = Not Equal?(x=w415, y=w413) -> (x != y?=w414:bool)
            n165 = case shown="True" w414 {
              tunnel: [w424 w425] -> w420
              tunnel: w417 -> [w423 w425]
              tunnel: w416 -> [w422 _]
              tunnel: w413 -> [w421 _]
              frame True {
                n166 = invoke class="VI" method="FP.Open"(reference=w422, error in=w423, "State"=w421) -> (error out=w424:errorcluster)  [unwired: 2 in, 4 out]
              }
              frame False {
              }
            }
          }
          frame "Minimize", "Minimized" {
            w426 = T8."Minimized" ("State")
            n167 = property class="VI"(reference=w432, error in=w431) -> (reference out=w429:refnum<vi>, error out=w430:errorcluster, "FP.State"=w428:T8)
            n168 = Not Equal?(x=w428, y=w426) -> (x != y?=w427:bool)
            n169 = case shown="True" w427 {
              tunnel: [w437 w438] -> w433
              tunnel: w430 -> [w436 w438]
              tunnel: w429 -> [w435 _]
              tunnel: w426 -> [w434 _]
              frame True {
                n170 = invoke class="VI" method="FP.Open"(reference=w435, error in=w436, "State"=w434) -> (error out=w437:errorcluster)  [unwired: 2 in, 4 out]
              }
              frame False {
              }
            }
          }
          frame "Maximize", "Maximized" {
            w439 = T8."Maximized" ("State")
            n171 = property class="VI"(reference=w445, error in=w444) -> (reference out=w442:refnum<vi>, error out=w443:errorcluster, "FP.State"=w441:T8)
            n172 = Not Equal?(x=w441, y=w439) -> (x != y?=w440:bool)
            n173 = case shown="True" w440 {
              tunnel: [w450 w451] -> w446
              tunnel: w443 -> [w449 w451]
              tunnel: w442 -> [w448 _]
              tunnel: w439 -> [w447 _]
              frame True {
                n174 = invoke class="VI" method="FP.Open"(reference=w448, error in=w449, "State"=w447) -> (error out=w450:errorcluster)  [unwired: 2 in, 4 out]
              }
              frame False {
              }
            }
          }
        }
        n175 = call <vilib>:"Add State(s) to Queue__JKI_lib_State_Machine.vi"("State(s) in (\"\")"=w386) -> ("States Out"=w385:string)  [unwired: 14 in]
      }
      frame "UI: Update Broadcast Registry" {
        n176 = call "CSM - List Mapping Relationships in Broadcast Registry.vi"() -> ("Mapping Relationships"=w453:T15)  [unwired: 10 in, 1 out]
        n177 = for {
          tunnel: w453 -> [w466] mode=indexing
          tunnel: [w459] -> w454 mode=indexing
          n178 = Unbundle(w466) -> (w465:string, "Name"=w464:string, "Target CSM"=w463:string, "Target State"=w462:string, "Register Type"=w461:T14)
          n179 = Format Into String(w461) -> (resulting string=w460:string)  [unwired: 3 in, 1 out]
          n180 = Build Array(w465, w464, w463, w462, w460) -> (w459:string[])
        }
        "Broadcast Registry" <- w454
      }
      frame "UI: Update Toolbar" {
        w475 = i16 2 ("x")
        n181 = control-ref of="Record.Start"() -> (w483:refnum<vi>)
        n182 = control-ref of="Record.Stop"() -> (w482:refnum<vi>)
        n183 = Unbundle By Name(w481) -> ("Core.Current VI Reference"=w472:refnum<vi>, "LogFile"=w469:path, "LoggerWatchDogQueue"=w480:refnum<queue>)
        n184 = Not A Number/Path/Refnum?(number/path/refnum=w480) -> (NaN/Path/Refnum?=w473:bool)
        n185 = Not(x=w473) -> (.not. x?=w474:bool)
        n186 = Boolean To (0,1)(Boolean=w474) -> (0, 1=w479:i16)
        n187 = Boolean To (0,1)(Boolean=w473) -> (0, 1=w478:i16)
        n188 = Multiply(x=w475, y=w478) -> (x*y=w476:i16)
        n189 = Multiply(x=w475, y=w479) -> (x*y=w477:i16)
        n190 = Empty String/Path?(string/path=w469) -> (empty?=w468:bool)
        n191 = property class="Bool"(reference=w483, "DisabledEnum"=w477) -> ()  [unwired: 1 in, 2 out]
        n192 = property class="Bool"(reference=w482, "DisabledEnum"=w476) -> ()  [unwired: 1 in, 2 out]
        n193 = case shown="True" w468 {
          tunnel: "Running Log Viewer (CSM)" ("Front Panel Window:Title") -> [w491 w492]
          tunnel: [w490 w492] -> w470
          tunnel: w469 -> [w487 _]
          frame False {
            n194 = Path To String(path=w487) -> (string=w488:string)
            n195 = Concatenate Strings(w491, " - " ("string"), w488) -> (w490:string)
          }
          frame True {
          }
        }
        n196 = property class="VI"(reference=w472, "Front Panel.Title"=w470) -> ()  [unwired: 1 in, 2 out]
      }
      frame "UI: Resize Tab Content" {
        n197 = control-ref of="Tab"() -> (w499:refnum<vi>)
        n198 = invoke class="TabCtl (strict)" method="FitControlToPane"(reference=w499) -> (reference out=w495:refnum<vi>, error out=w493:errorcluster)  [unwired: 2 in, 1 out]
        n199 = control-ref of="Error History"() -> (w497:refnum<vi>)
        n200 = control-ref of="State History"() -> (w496:refnum<vi>)
        n201 = control-ref of="Broadcast Registry"() -> (w498:refnum<vi>)
        n202 = Build Array(w498, w497, w496) -> (w494:refnum<vi>[])
        n203 = for {
          tunnel: w495 -> [w507]
          tunnel: w494 -> [w506] mode=indexing
          tunnel: w493 -> [w505]
          n204 = call "Fit Control to Tab.vi"("Control"=w506, "error in (no error)"=w505, "TabRef"=w507) -> ()  [unwired: 5 in, 2 out]
        }
      }
      frame "---------- Macro ----------" {
        # "Do not put any code in this frame.\n(It is a separator no-op. You can make a copy of this frame to create a new Macro frame)"
        n205 = call <vilib>:"Add State(s) to Queue__JKI_lib_State_Machine.vi"("State(s) in (\"\")"=w513) -> ("States Out"=w512:string)  [unwired: 14 in]
      }
      frame "Macro: Initialize" {
        w516 = "Data: Initialize\nData: Initialize References\nInitialize Core Data\nUI: Initialize\nUI: Front Panel State >> Open\nUI: Resize Tab Content\nUI: Update Broadcast Registry\nUI: Update Toolbar"  # Data: Initialize Data: Initialize References Initialize Core Data UI: Initialize UI: Front Panel State >> Open UI: Resize Tab Content UI: Update Broadcast Registry UI: Update Toolbar
        # "Initialization Macro\n(This is called once, when the VI starts)"
        n206 = call <vilib>:"Add State(s) to Queue__JKI_lib_State_Machine.vi"("State(s) in Front (\"\")"=w516, "State(s) in (\"\")"=w520) -> ("States Out"=w519:string)  [unwired: 13 in]
      }
      frame "Macro: Exit" {
        (unwired) ""
        # "Exit Macro\n(This is called once, when the VI exits)"
        n207 = Unbundle By Name(w525) -> ()  [unwired: 1 out]
        n208 = call <vilib>:"Add State(s) to Queue__JKI_lib_State_Machine.vi"("State(s) at Back (\"\")"="Data: Cleanup\nExit") -> ("States Out"=w523:string)  [unwired: 14 in]
        n209 = call <vilib>:"Add State(s) to Queue__JKI_lib_State_Machine.vi"("State(s) in Front (\"\")"=w523, "State(s) in (\"\")"=w528) -> ("States Out"=w527:string)  [unwired: 13 in]
      }
    }
  }
  n210 = disable-structure shown="Disabled" {
    frame Disabled {
      n211 = call "CSM - Module VI Reference.vi"("Response Timeout (-2 Using Global Settings)"=1000 ("Response Timeout(5000 ms)"), "error in (no error)"=errorcluster {"status"=FALSE, "code"=0, "source"=""}, "CSM Name"="") -> ("error out"=w535:errorcluster, "CSM Module VIRef"=w534:refnum<vi>)  [unwired: 7 in]
      n212 = invoke on="Invoke Node" class="VI" method="FP.Open"(reference=w534, error in=w535, "Activate"=TRUE ("Activate?")) -> (error out=w533:errorcluster)  [unwired: 2 in, 4 out]
      n213 = call <vilib>:"Simple Error Handler.vi"("error in (no error)"=w533) -> ()  [unwired: 4 in, 5 out]
    }
    frame Enabled {
    }
  }
  n214 = flat-sequence {
    tunnel: [w537] -> w8
    tunnel: w7 -> [w537]
    frame #0 {
      n215 = local write "Stop"(TRUE ("Stop")) -> ()
    }
  }
  n216 = call "CSM - Destroy Global Log Queue.vi"("Error In"=w17, "Global Log Queue"=w15) -> ("error out"=w9:errorcluster)  [unwired: 9 in]
  n217 = control-ref of="Current VI Reference"() -> (w4:refnum<vi>)
  n218 = Merge Errors(w8, w9) -> (w2:errorcluster)
  n219 = call "Close FP if in LabVIEW Dir.vi"("VI Refnum"=w4, "Error in"=w2) -> ("Error out"=w5:errorcluster)  [unwired: 9 in]
  n220 = call <vilib>:"Clear Errors.vi"("error in (no error)"=w5) -> ()  [unwired: 5 in, 2 out]
